vi "set_open_circuit.vi"(8 "error in (no error)":errorcluster, 11 "VISA Refnum in":refnum<visa-resource-name>) -> (0 "error out":errorcluster, 3 "VISA Refnum out":refnum<visa-resource-name>)   [LabVIEW 2018]
uses:
  <instrlib>/Keithley 24XX/Keithley 24XX.lvlib
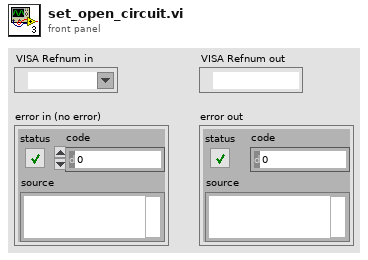
[diagram p1: front panel]
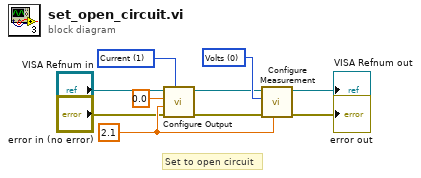
[diagram p0: block diagram]
diagram:
  w10 = 2.1 ("Compliance  Level (0.1)")
  w9 = u16 0 items=["Volts", "Current", "Resistance"] ("Function (0: Volts)")
  w8 = u16 1 items=["Voltage", "Current"] ("Source Mode  (0: Voltage)")
  # "Set to open circuit"
  n1 = call <instrlib>:"Configure Output.vi"("Source Mode  (0: Voltage)"=w8, "error in (no error)"="error in (no error)", "Compliance  Level (0.1)"=w10, "Output Level (0)"=0.0, "VISA resource name"="VISA Refnum in") -> ("error out"=w2:errorcluster, "VISA resource name out"=w1:refnum<visa-resource-name>)  [unwired: 1 in, 4 out]
  n2 = call <instrlib>:"Configure Measurement.vi"("Manual Range (1.0)"=w10, "error in (no error)"=w2, "Function (0: Volts)"=w9, "VISA resource name"=w1) -> ("error out"=→"error out":errorcluster, "VISA resource name out"=→"VISA Refnum out":refnum<visa-resource-name>)  [unwired: 1 in, 5 out]
